vi "Get Session Handle.vi"(8 "Error In":errorcluster, 11 "object in":refnum<class "Pulsetrain Config.lvclass">=refnum) -> (0 "Error Out":errorcluster, 2 "Session Handle":refnum<k15>, 3 "object out":refnum<class "Pulsetrain Config.lvclass">)   [LabVIEW 2023, in "Teledyne-T3AFG120.lvlib" / "Pulsetrain Config.lvclass"]
uses:
  Pulsetrain Config.lvclass
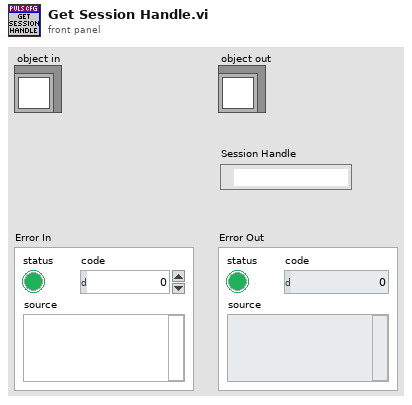
[diagram p1: front panel]
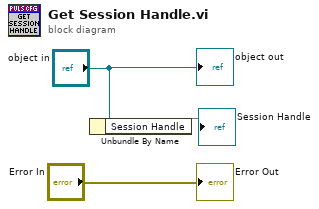
[diagram p0: block diagram]
diagram:
  n1 = Unbundle By Name("object in") -> ("Session Handle"=→"Session Handle")
  "Error Out" <- "Error In"
  "object out" <- "object in"
